vi "PUT (File).vi"(6 "timeout":i32=10000, 7 "output file":path, 8 "error in":errorcluster, 9 "file":path, 10 "url":string, 11 "session in":refnum<class "Session.lvclass">) -> (0 "error out":errorcluster, 1 "body":string, 2 "headers":string, 3 "session out":refnum<class "Session.lvclass">, 4 "status code":u32)   [LabVIEW 2024, in "lib_NI_Advanced HTTP Client.lvlib" / "Session.lvclass"]
uses:
  Session.lvclass
  Session.lvclass/Session.ctl
  lvwebclient_64.dll
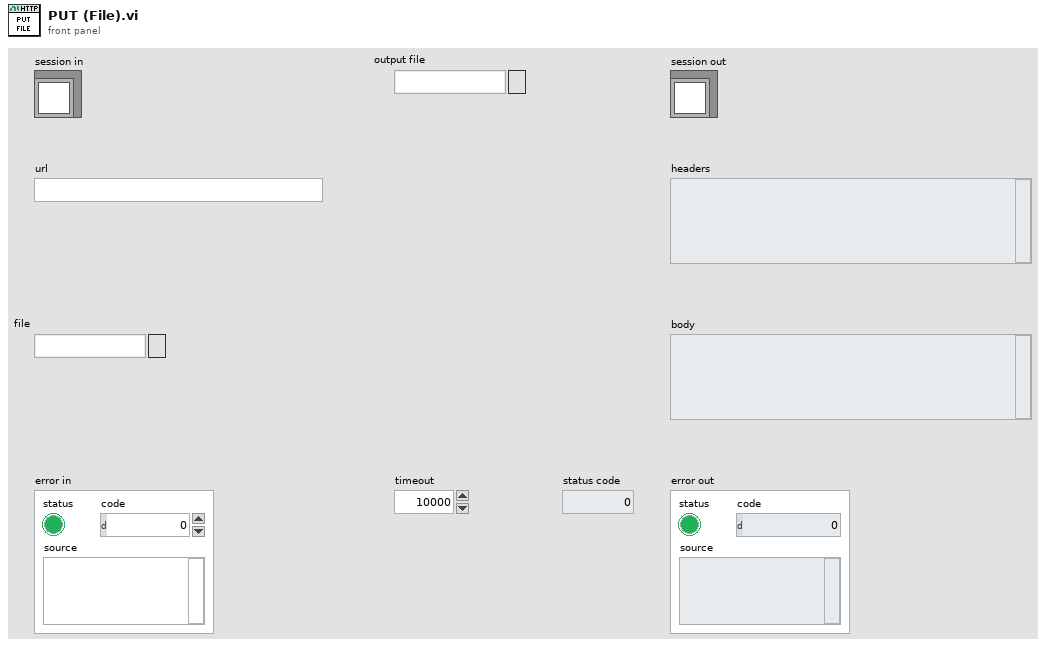
[diagram p1: front panel]
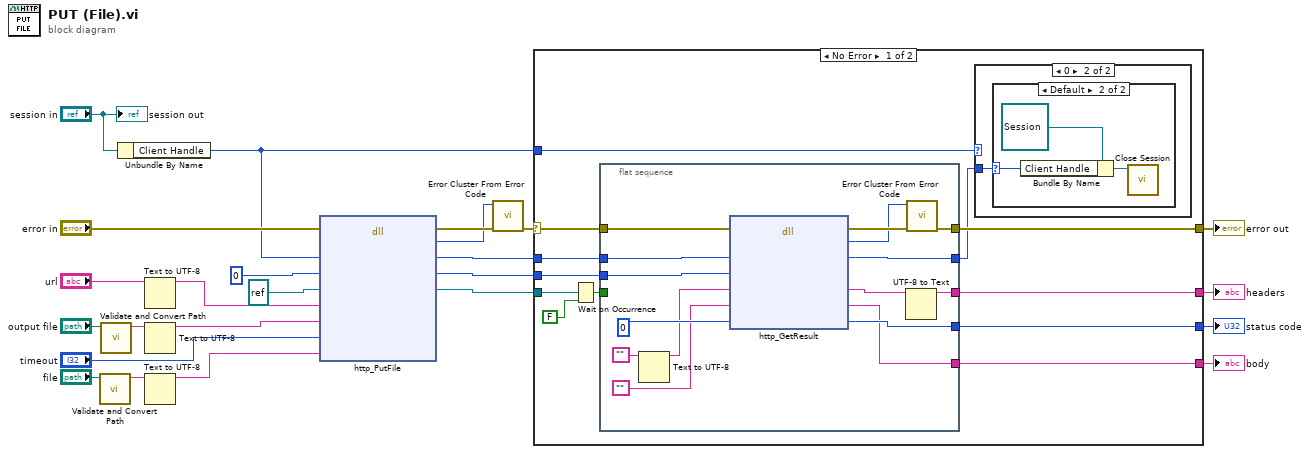
[diagram p0: block diagram]
diagram:
  n1 = call "Validate and Convert Path.vi"("path"="file") -> ("validated path as string"=w2:string)  [unwired: 10 in]
  n2 = call "Validate and Convert Path.vi"("path"="output file") -> ("validated path as string"=w16:string)  [unwired: 10 in]
  n3 = Unbundle By Name("session in") -> ("Client Handle"=w11:u32)
  n4 = Text to UTF-8(11:"url") -> (3:w5:string)  [unwired: 2 in, 1 out]
  n5 = Text to UTF-8(11:w16) -> (3:w4:string)  [unwired: 2 in, 1 out]
  n6 = Text to UTF-8(11:w2) -> (3:w1:string)  [unwired: 2 in, 1 out]
  n7 = dll-call lib="C:/Program Files/National Instruments/LabVIEW 2024/vi.lib/NI/Advanced HTTP Client/lvwebclient_*.*" fn="http_PutFile"(error in="error in", "handle"=w11, "request"=u32 0, "completeOccurrence"=refnum<k4> refnum ("occurrence"), "url"=w5, "outPath"=w4, "timeout"="timeout", "putFile"=w1) -> (error out=w13:errorcluster, "return"=w12:i32, "handle"=w8:u32, "request"=w7:u32, "completeOccurrence"=w6:refnum<k4>)  [unwired: 6 in, 1 out]
  n8 = call "Error Cluster From Error Code.vi"("error in (no error)"=w13, "error code (0)"=w12) -> ("error out"=w24:errorcluster)  [unwired: 7 in]
  n9 = case shown="No Error" w24 {
    selector: w24 -> [w34 w56]
    tunnel: w6 -> [w36 _]
    tunnel: w8 -> [w33 _]
    tunnel: w7 -> [w32 _]
    tunnel: [w31 _] -> w21
    tunnel: [w30 _] -> w20
    tunnel: [w29 _] -> w19
    tunnel: [w28 w56] -> w18
    tunnel: w11 -> [w27 _]
    frame No Error {
      n10 = Wait on Occurrence(1:FALSE, 2:w36) -> (0:w35:bool)  [unwired: 1 in]
      n11 = flat-sequence {
        tunnel: w35 -> [_]
        tunnel: w34 -> [w55]
        tunnel: w33 -> [w54]
        tunnel: w32 -> [w53]
        tunnel: [w51] -> w31
        tunnel: [w46] -> w30
        tunnel: [w47] -> w29
        tunnel: [w45] -> w28
        tunnel: [w44] -> w26
        frame #0 {
          n12 = Text to UTF-8(11:"") -> (3:w42:string)  [unwired: 2 in, 1 out]
          n13 = dll-call lib="C:/Program Files/National Instruments/LabVIEW 2024/vi.lib/NI/Advanced HTTP Client/lvwebclient_*.*" fn="http_GetResult"(error in=w55, "handle"=w54, "request"=w53, "returnHeader"=w42, "returnBody"="", "httpStatus"=u32 0) -> (error out=w50:errorcluster, "return"=w49:i32, "handle"=w44:u32, "returnHeader"=w48:string, "returnBody"=w47:string, "httpStatus"=w51:u32)  [unwired: 3 in, 1 out]
          n14 = UTF-8 to Text(11:w48) -> (3:w46:string)  [unwired: 2 in, 1 out]
          n15 = call "Error Cluster From Error Code.vi"("error in (no error)"=w50, "error code (0)"=w49) -> ("error out"=w45:errorcluster)  [unwired: 7 in]
        }
      }
      n16 = case shown="0" w27 {
        tunnel: w26 -> [_ w37]
        frame Default {
        }
        frame 0 {
          n17 = case shown="Default" w37 {
            selector: w37 -> [_ w40]
            frame 0 {
            }
            frame Default {
              n18 = Bundle By Name(cluster=refnum<class "Session.lvclass"> refnum ("NI_Advanced HTTP Client.lvlib:Session.lvclass"), "Client Handle"=w40) -> (w39:refnum<class "Session.lvclass">)
              n19 = call "Close Session.vi"("session"=w39) -> ()  [unwired: 10 in, 1 out]
            }
          }
        }
      }
    }
    frame Error {
    }
  }
  "error out" <- w18
  "headers" <- w20
  "body" <- w19
  "status code" <- w21
  "session out" <- "session in"
